vi "NovaTech409A_PowerToCommand.vi"(1 "Novatech Power [dBm]":dbl) -> (0 "Novatech Command":u16)   [LabVIEW 2013, in "Novatech 409A.lvlib"]
uses:
  Novatech 409A.lvlib
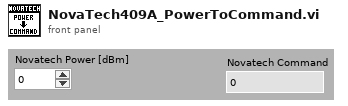
[diagram p1: front panel]
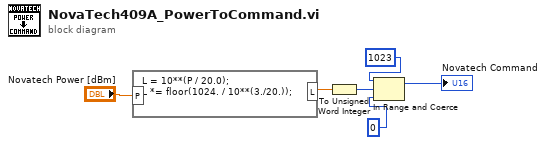
[diagram p0: block diagram]
diagram:
  n1 = formula code="L = 10**(P / 20.0);\nL *= floor(1024. / 10**(3./20.));"("P"="Novatech Power [dBm]") -> ("L"=w6:dbl)
  n2 = To Unsigned Word Integer(number=w6) -> (unsigned 16bit integer=w1:u16)
  n3 = In Range and Coerce(upper limit=u16 1023, x=w1, lower limit=u16 0) -> (coerced(x)=→"Novatech Command":u16)  [unwired: 1 out]
